vi "Day 03 Part 1.vi"(11 "Input":string) -> (3 "Output":u32)   [LabVIEW 2021]
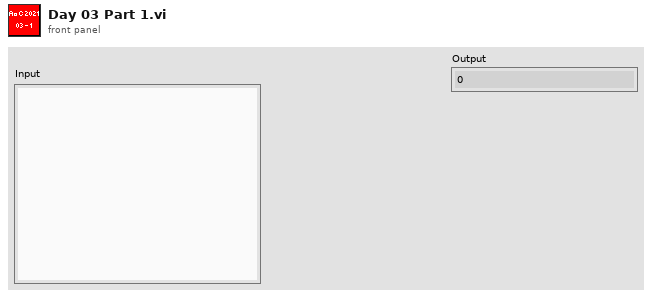
[diagram p1: front panel]
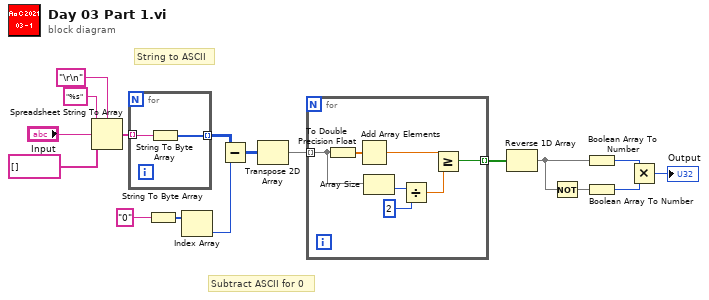
[diagram p0: block diagram]
diagram:
  # "Subtract ASCII for 0"
  # "String to ASCII"
  n1 = Spreadsheet String To Array(delimiter (Tab)="\r\n", format string="%s", spreadsheet string="Input", array type (2D Dbl)=string[] []) -> (array=w14:string[])
  n2 = for {
    tunnel: w14 -> [w19] mode=indexing
    tunnel: [w18] -> w5 mode=indexing
    n3 = String To Byte Array(string=w19) -> (unsigned byte array=w18:u8[])
  }
  n4 = String To Byte Array(string="0" ("delimiter (Tab)")) -> (unsigned byte array=w12:u8[])
  n5 = Index Array(array=w12) -> (element=w7:u8)  [unwired: 1 in]
  n6 = Subtract(x=w5, y=w7) -> (x-y=w6:u8[][])
  n7 = Transpose 2D Array(2D array=w6) -> (transposed array=w10:u8[][])
  n8 = for {
    tunnel: w10 -> [w20] mode=indexing
    tunnel: [w22] -> w9 mode=indexing
    n9 = To Double Precision Float(number=w20) -> (double precision float=w21:dbl[])
    n10 = Add Array Elements(numeric array=w21) -> (sum=w24:dbl)
    n11 = Array Size(array=w20) -> (size(s)=w26:i32)
    n12 = Divide(x=w26, y=2) -> (x/y=w23:dbl)
    n13 = Greater Or Equal?(x=w24, y=w23) -> (x >= y?=w22:bool)
  }
  n14 = Reverse 1D Array(array=w9) -> (reversed array=w2:bool[])
  n15 = Not(x=w2) -> (.not. x?=w1:bool[])
  n16 = Boolean Array To Number(Boolean array=w2) -> (number=w3:u32)
  n17 = Boolean Array To Number(Boolean array=w1) -> (number=w4:u32)
  n18 = Multiply(x=w3, y=w4) -> (x*y=→"Output":u32)
